vi "check.file.last_update.vi"(8 "error in (no error)":errorcluster, 11 "comic_crawler in":refnum<class "comic_crawler.lvclass">) -> (0 "error out":errorcluster, 3 "comic_crawler out":refnum<class "comic_crawler.lvclass">)   [LabVIEW 2024, in "comic_crawler.lvclass"]
uses:
  comic_crawler.lvclass
  comic_crawler.lvclass/comic_crawler.ctl
  WebScraper/comic_class/comic_class.lvclass/comic_class.ctl
  WebScraper/comic_class/comic_class.lvclass
  <vilib>/addons/_JKI.lib/Serialization/JSON/JKI JSON Serialization.lvlib
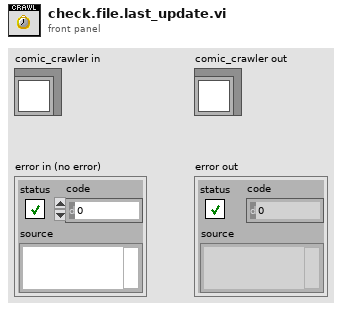
[diagram p1: front panel]
types:
  T1 = cluster{"date_last_updated":timestamp, "site_detail_url":string, "sortable_name":string}
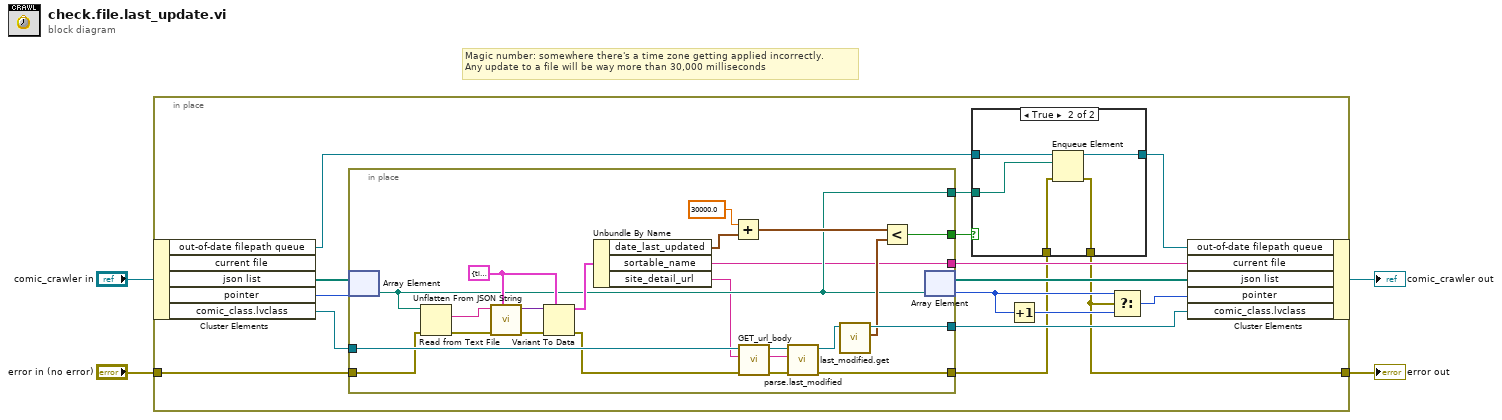
[diagram p0: block diagram]
diagram:
  # "Magic number: somewhere there's a time zone getting applied incorrectly.\nAny update to a file will be way more than 30,000 milliseconds"
  n1 = in-place {
    in-place-border: "error in (no error)" -> [w16]
    in-place-border: [w5] -> w1
    n2 = in-place-cluster #1("comic_crawler in") -> ("out-of-date filepath queue"=w10:refnum<queue>, "json list"=w20:path[], "pointer"=w19:i32, "comic_class.lvclass"=w18:refnum<class "comic_class.lvclass">)  [unwired: 1 out]
    n3 = in-place {
      in-place-border: [w23] -> w11
      in-place-border: w18 -> [w34]
      in-place-border: [w33] -> w17
      in-place-border: w16 -> [w31]
      in-place-border: [w29] -> w6
      in-place-border: [w25] -> w8
      in-place-border: [w24] -> w7
      w39 = T1 {"date_last_updated"=timestamp(0 s since 1904-01-01), "site_detail_url"="", "sortable_name"=""}
      n4 = in-place-array #2(w20, w19) -> (w25:path)
      n5 = Read from Text File(file (use dialog)=w25, error in=w31) -> (text=w41:string, error out=w40:errorcluster)  [unwired: 2 in, 2 out]
      n6 = call <vilib>:"Unflatten From JSON String.vi"("Type and Defaults"=w39, "error in"=w40, "JSON String"=w41) -> ("error out"=w43:errorcluster, "Variant"=w42:variant)  [unwired: 7 in]
      n7 = Variant To Data(error in=w43, type=w39, Variant=w42) -> (data=w38:T1, error out=w32:errorcluster)
      n8 = Unbundle By Name(w38) -> ("date_last_updated"=w22:timestamp, "sortable_name"=w23:string, "site_detail_url"=w21:string)
      n9 = Add(x=30000.0 ("y"), y=w22) -> (x+y=w27:timestamp)
      n10 = call-dynamic "GET_url_body.vi"("error in (no error)"=w32, "url"=w21, "comic_class in"=w34) -> ("error out"=w30:errorcluster, "body"=w36:string, "comic_class out"=w35:refnum<class "comic_class.lvclass">)  [unwired: 6 in]
      n11 = call-dynamic "parse.last_modified.vi"("error in (no error)"=w30, "body"=w36, "comic_class in"=w35) -> ("error out"=w29:errorcluster, "comic_class out"=w37:refnum<class "comic_class.lvclass">)  [unwired: 7 in]
      n12 = call "last_modified.get.vi"("comic_class in"=w37) -> ("last modified"=w26:timestamp, "comic_class out"=w33:refnum<class "comic_class.lvclass">)  [unwired: 9 in]
      n13 = Less?(x=w27, y=w26) -> (x < y?=w24:bool)
      n14 = in-place-array #2(w25) -> (w15:path[], w13:i32)
    }
    n15 = case shown="True" w7 {
      tunnel: w10 -> [w45 w50]
      tunnel: [w45 w49] -> w9
      tunnel: w8 -> [_ w48]
      tunnel: w6 -> [w44 w47]
      tunnel: [w44 w46] -> w5
      frame False {
      }
      frame True {
        n16 = Enqueue Element(queue=w50, element=w48, error in (no error)=w47) -> (queue out=w49:refnum<queue>, error out=w46:errorcluster)  [unwired: 1 in, 1 out]
      }
    }
    n17 = Increment(x=w13) -> (x+1=w12:i32)
    n18 = Select(t=w13, s=w5, f=w12) -> (s? t:f=w14:i32)
    n19 = in-place-cluster #1("out-of-date filepath queue"=w9, "current file"=w11, "json list"=w15, "pointer"=w14, "comic_class.lvclass"=w17) -> (→"comic_crawler out":refnum<class "comic_crawler.lvclass">)
  }
  "error out" <- w1
